vi "Array Days Of The Week Continued.vi"() -> ()   [LabVIEW 2012]
panel:
  out "Week Day":string
  out "Range Of Days":string[](array[string])
  in  "Sub Range Length":dbl(knob)=4.0 min=0.0 max=7.0 step=1.0 scale=0.0..7.0
  in  "Select Week Day":dbl(knob)=2.0 min=0.0 max=6.0 step=1.0 scale=0.0..6.0
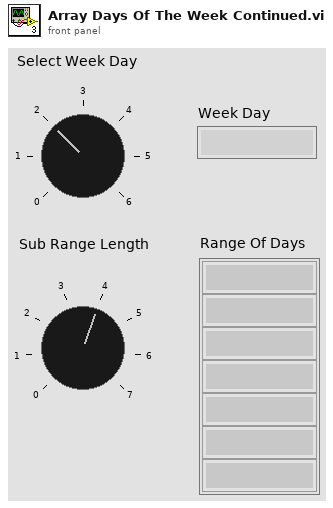
[diagram p1: front panel]
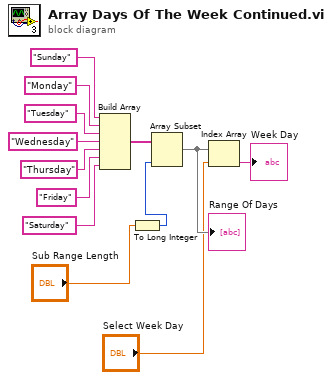
[diagram p0: block diagram]
diagram:
  n1 = Build Array("Sunday", "Monday", "Tuesday", "Wednesday", "Thursday", "Friday", "Saturday") -> (w3:string[])
  n2 = To Long Integer(number="Sub Range Length") -> (32bit integer=w1:i32)
  n3 = Array Subset(array=w3, length=w1) -> (w12:string[])  [unwired: 1 in]
  "Range Of Days" <- w12
  n4 = Index Array(array=w12, index="Select Week Day") -> (element=→"Week Day":string)
